vi "Create Control Ref Endpoint.vi"(3 "Bundler Terminal":refnum<vi>, 8 "Terminal Config":T1, 9 "Terminal":refnum<vi>, 10 "Frames[]":refnum<vi>[](array[refnum]), 11 "Index":i32) -> (0 "error out":errorcluster)   [LabVIEW 2020, in "FlexBlocks.lvlib"]
uses:
  FlexBlocks.lvlib
  Terminal Config.ctl
  Type Descriptor.ctl
  Terminal Direction.ctl
  Value Mode.ctl
  Special Terminal.ctl
  Terminal Mode.ctl
  <vilib>/Utility/miscctls.llb/LVPointTypeDef.ctl
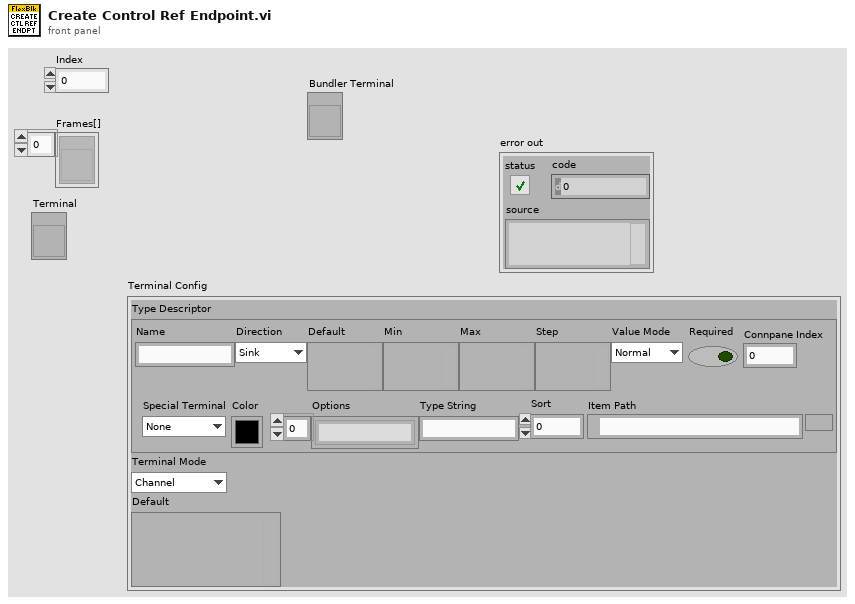
[diagram p1: front panel]
types:
  T1 = typedef "FlexBlocks.lvlib/Terminal Config.ctl" = cluster{"Type Descriptor":T2, "Terminal Mode":T6, "Default":variant}
  T2 = typedef "FlexBlocks.lvlib/Type Descriptor.ctl" = cluster{"Name":string, "Direction":T3, "Default":variant, "Min":variant, "Max":variant, "Step":variant, "Value Mode":T4, "Required":bool, "Connpane Index":i32, "Special Terminal":T5, "Color":u32, "Options":string[], "Type String":string, "Sort":i32, "Item Path":path}
  T3 = typedef "FlexBlocks.lvlib/Terminal Direction.ctl" = enum16{"Sink", "Source"}
  T4 = typedef "FlexBlocks.lvlib/Value Mode.ctl" = enum16{"Normal", "Range", "Select"}
  T5 = typedef "FlexBlocks.lvlib/Special Terminal.ctl" = enum16{"None", "Action", "Init", "Tag", "State in", "State out", "Error"}
  T6 = typedef "FlexBlocks.lvlib/Terminal Mode.ctl" = enum16{"Channel", "Config", "Value", "Control Ref"}
  T7 = typedef "LVPointTypeDef.ctl" = cluster{"Horizontal":i16, "Vertical":i16}
  T8 = typedef "FlexBlocks.lvlib/Paths.ctl" = cluster{"FlexBlocks":path, "Workers Root":path, "Specialized Editors":path, "Worker Template":path, "Editor Template":path, "Express Template":path, "Control Ref Vim":path}
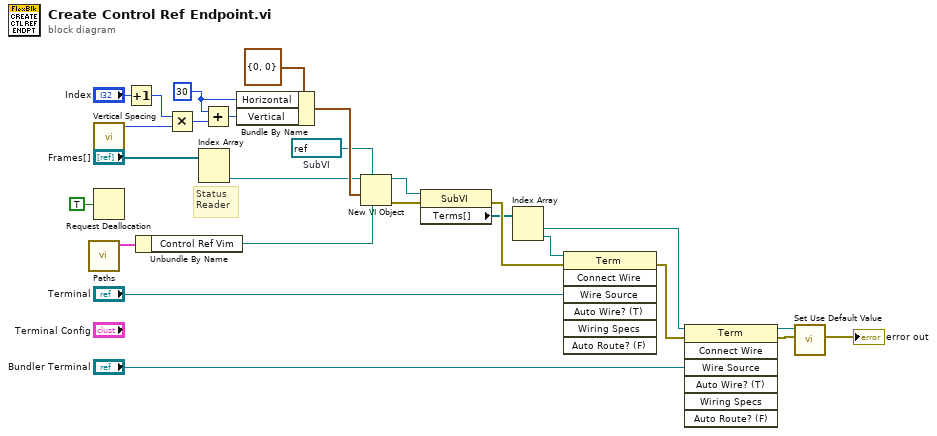
[diagram p0: block diagram]
diagram:
  w10 = 30 ("Left")
  w16 = refnum<vi> refnum  # SubVI
  # "Status\nReader"
  n1 = call "Paths.vi"() -> ("Paths"=w6:T8)  [unwired: 11 in]
  n2 = call "Vertical Spacing.vi"() -> ("Spacing"=w18:i32)  [unwired: 11 in]
  n3 = Request Deallocation(TRUE ("flag")) -> ()
  n4 = Increment(x="Index") -> (x+1=w20:i32)
  n5 = Unbundle By Name(w6) -> ("Control Ref Vim"=w5:path)
  n6 = Multiply(x=w20, y=w18) -> (x*y=w12:i32)
  n7 = Index Array(array="Frames[]") -> (element #2=w19:refnum<vi>)  [unwired: 2 in, 1 out]
  n8 = Add(x=w10, y=w12) -> (x+y=w11:i32)
  n9 = Bundle By Name(cluster=T7 {"Horizontal"=0, "Vertical"=0} ("location"), "Horizontal"=w10, "Vertical"=w11) -> (w26:T7)
  n10 = New VI Object(vi object class=w16, owner refnum=w19, position/next to=w26, 6:w5) -> (object refnum=w15:refnum<vi>, 0:w25:errorcluster)  [unwired: 4 in]
  n11 = property class="SubVI"(reference=w15, error in=w25) -> (error out=w24:errorcluster, "Terms[]"=w14:refnum<vi>[])  [unwired: 1 out]
  n12 = Index Array(array=w14) -> (element #1=w7:refnum<vi>, element #2=w8:refnum<vi>)  [unwired: 2 in]
  n13 = invoke class="Term" method="Connect Wire"(reference=w8, error in=w24, "Wire Source"="Terminal") -> (error out=w4:errorcluster)  [unwired: 4 in, 6 out]
  n14 = invoke class="Term" method="Connect Wire"(reference=w7, error in=w4, "Wire Source"="Bundler Terminal") -> (reference out=w3:refnum<vi>, error out=w2:errorcluster)  [unwired: 4 in, 5 out]
  n15 = call "Set Use Default Value.vi"("error in (no error)"=w2, "Terminal"=w3) -> ("error out"=→"error out":errorcluster)  [unwired: 9 in]
